vi "Out Of Band Communication.vi"(6 "gRPC to Main":T3, 7 "State In":T1=enum."Execute Logic", 8 "error in":errorcluster, 11 "Node in":refnum<class "AMS Climate Chamber Template.lvclass">) -> (0 "error out":errorcluster, 1 "Update Local Variable":bool, 3 "Node out":refnum<class "AMS Climate Chamber Template.lvclass">, 4 "Main to gRPC":T2, 5 "State Out":T1=enum."Execute Logic")   [LabVIEW 2023, in "AMS Climate Chamber Template.lvlib" / "AMS Climate Chamber Template.lvclass"]
uses:
  AMS Climate Chamber Template.lvclass
  Out Of Band/Type Defs/gRPC to Main.ctl
  Out Of Band/Type Defs/Main to gRPC.ctl
  <vilib>/ADAS Replay HIL/ADAS Plugin Utilities/AdasLvTemplate/Typedefs/Default Plug-in States.ctl
  Out Of Band/Main Loop/Class to Main_to_gRPC.vi
  <vilib>/ADAS Replay HIL/ADAS Plugin Utilities/AdasLvTemplate/AdasLvTemplate.lvclass
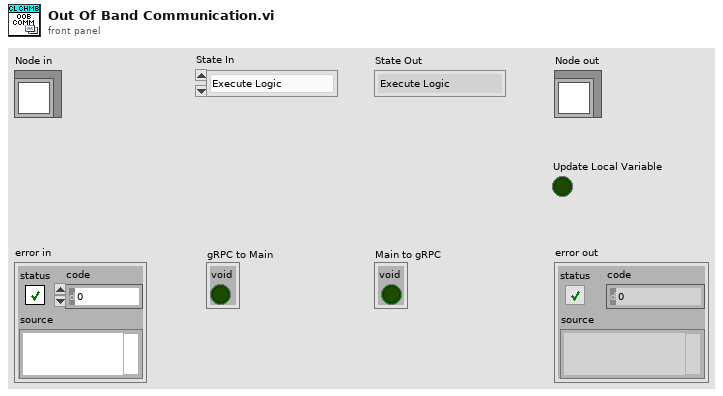
[diagram p1: front panel]
types:
  T1 = typedef "AdasLvTemplate.lvlib/AdasLvTemplate.lvclass/Default Plug-in States.ctl" = enum16{"Start", "Pause", "Restart", "Execute Logic", "Housekeeping", "Error", "Shutdown"}
  T2 = typedef "AMS Climate Chamber Template.lvlib/AMS Climate Chamber Template.lvclass/Main to gRPC.ctl" = cluster{"void":bool}
  T3 = typedef "AMS Climate Chamber Template.lvlib/AMS Climate Chamber Template.lvclass/gRPC to Main.ctl" = cluster{"void":bool}
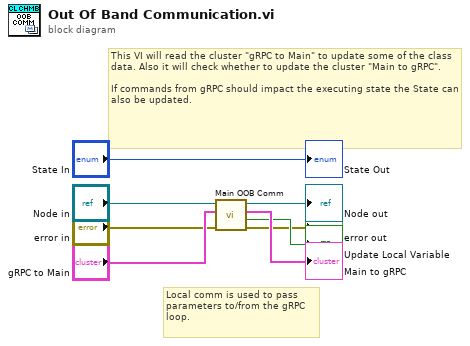
[diagram p0: block diagram]
diagram:
  # "This VI will read the cluster \"gRPC to Main\" to update some of the class data. Also it will check whether to update the cluster \"Main to gRPC\".\n\nIf commands from gRPC should impact the executing state the State can also be updated."
  # "Local comm is used to pass parameters to/from the gRPC loop."
  n1 = call "Main OOB Comm.vi"("error in"="error in", "gRPC to Main"="gRPC to Main", "Node in"="Node in") -> ("error out"=→"error out":errorcluster, "Update"=→"Update Local Variable":bool, "Main to gRPC"=→"Main to gRPC":T2, "Node out"=→"Node out":refnum<class "AMS Climate Chamber Template.lvclass">)  [unwired: 5 in]
  "State Out" <- "State In"
